vi "Create Reservation Observer.vi"(8 "error in":errorcluster, 10 "measurement context":refnum<class "MeasurementContext.lvclass">) -> (0 "error out":errorcluster, 3 "reservation observer out":refnum<class "Reservation Observer.lvclass">)   [LabVIEW 2020, in "MeasurementLink Measurement Server.lvlib" / "Reservation Observer.lvclass"]
uses:
  Reservation Observer.lvclass
  Reservation Observer.lvclass/Reservation Observer.ctl
  Classes/MeasurementContext/MeasurementContext.lvclass
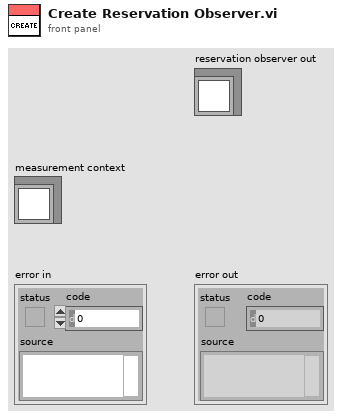
[diagram p1: front panel]
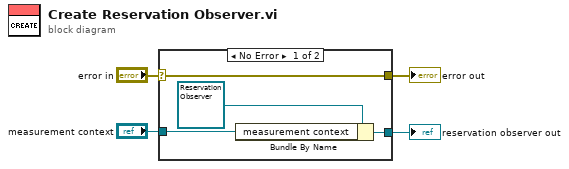
[diagram p0: block diagram]
diagram:
  n1 = case shown="No Error" "error in" {
    selector: "error in" -> [w8 w9]
    tunnel: [w8 w9] -> w3
    tunnel: [w6 _] -> w2
    tunnel: "measurement context" -> [w5 _]
    frame No Error {
      n2 = Bundle By Name(cluster=refnum<class "Reservation Observer.lvclass"> refnum ("Reservation Observer out"), "measurement context"=w5) -> (w6:refnum<class "Reservation Observer.lvclass">)
    }
    frame Error {
    }
  }
  "error out" <- w3
  "reservation observer out" <- w2
